vi "Write parallax_Arcsec.vi"(8 "error in (no error)":errorcluster, 10 "parallax_Arcsec":dbl[unit] min=0.0 max=4.84813681109536e-05, 11 "FixedTarget in":refnum<class "FixedTarget.lvclass">) -> (0 "error out":errorcluster, 3 "FixedTarget out":refnum<class "FixedTarget.lvclass">)   [LabVIEW 2014, in "TCSDataDefinitions.lvlib" / "TCSCommand.lvlib" / "TargetConfiguration.lvlib" / "Target.lvlib" / "FixedTarget.lvlib" / "FixedTarget.lvclass"]
uses:
  FixedTarget.lvclass
  FixedTarget.lvclass/FixedTarget.ctl
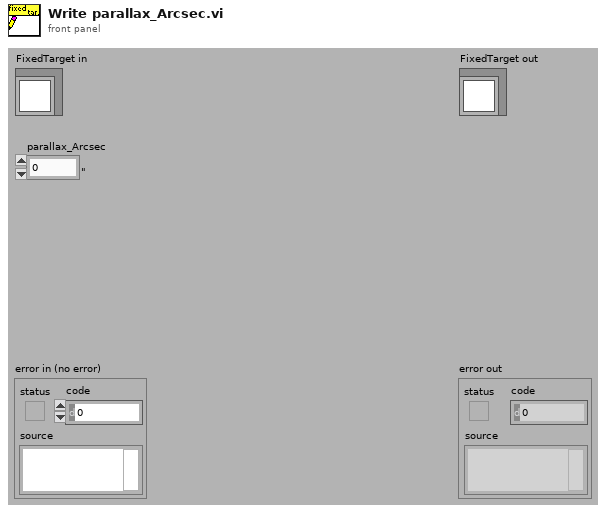
[diagram p1: front panel]
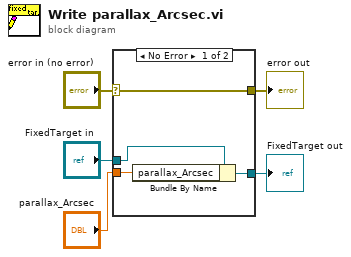
[diagram p0: block diagram]
diagram:
  n1 = case shown="No Error" "error in (no error)" {
    selector: "error in (no error)" -> [w9 w10]
    tunnel: [w9 w10] -> w4
    tunnel: [w7 w11] -> w2
    tunnel: "FixedTarget in" -> [w8 w11]
    tunnel: "parallax_Arcsec" -> [w6 _]
    frame No Error {
      n2 = Bundle By Name(cluster=w8, "parallax_Arcsec"=w6) -> (w7:refnum<class "FixedTarget.lvclass">)
    }
    frame Error {
    }
  }
  "error out" <- w4
  "FixedTarget out" <- w2
